vi "get_data.vi"(11 "file (use dialog)":path) -> (2 "Data Size":i32, 3 "Raw Data":dbl[](array[numeric]))   [LabVIEW 2018]
panel:
  out "text":string
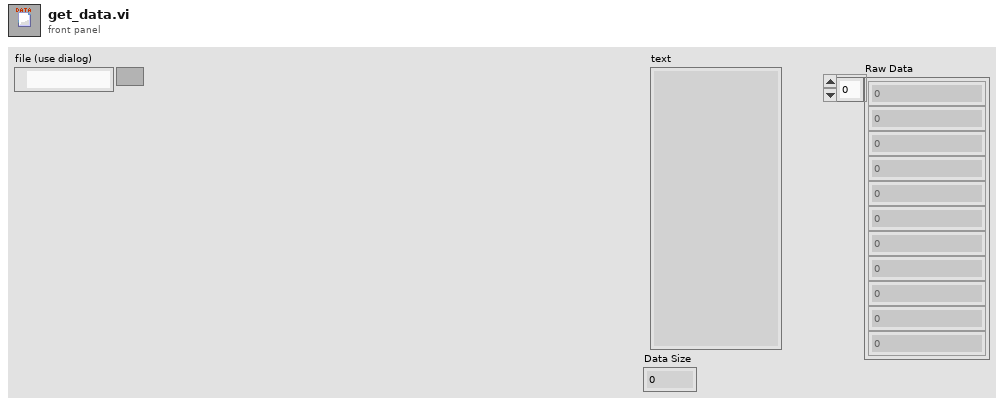
[diagram p1: front panel]
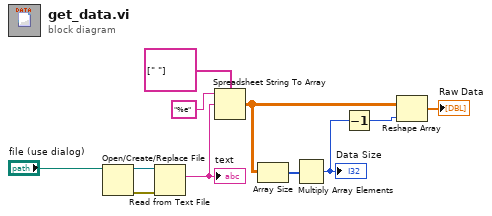
[diagram p0: block diagram]
diagram:
  n1 = Open/Create/Replace File(file path (use dialog)="file (use dialog)") -> (refnum out=w9:refnum<file>, error out=w10:errorcluster)  [unwired: 5 in, 1 out]
  n2 = Read from Text File(file (use dialog)=w9, error in=w10) -> (text=w8:string)  [unwired: 2 in, 3 out]
  "text" <- w8
  n3 = Spreadsheet String To Array(delimiter (Tab)=string[] [" "], format string="%e", spreadsheet string=w8) -> (array=w4:dbl[][])  [unwired: 1 in]
  n4 = Array Size(array=w4) -> (size(s)=w3:i32[])
  n5 = Multiply Array Elements(1:w3) -> (0:w2:i32)
  "Data Size" <- w2
  n6 = Decrement(x=w2) -> (x-1=w1:i32)
  n7 = Reshape Array(w4, w1) -> (→"Raw Data":dbl[])
